vi "Counter_BufferedPulseWidthMeasurement.vi"() -> ()   [LabVIEW 2020]
uses:
  <userlib>/DAQNavi Polymorphic VI/create/DAQNavi Create Channel(Buffered-CI-PulseWidth).vi
  <userlib>/DAQNavi Polymorphic VI/configure/timing/DAQNavi Timing(Buffered Counter Input).vi
  <userlib>/DAQNavi Polymorphic VI/configure/DAQNavi Get Property/CI/DAQNaviGet_Buffered_CI_Record_SectionCount.vi
  <userlib>/DAQNavi Polymorphic VI/read/DAQNavi Read (Buffered Counter Pulse Width).vi
  <userlib>/DAQNavi Polymorphic VI/configure/DAQNavi Get Property/CI/DAQNaviGet_Buffered_CI_Trigger_Level.vi
panel:
  out "data":cluster{"high period":dbl, "low period":dbl}[][](array[cluster])
  out "stopped?":bool
  in  "time out":dbl
  in  "number of samples per channel to read":u32=1000
  out "actual trigger level":dbl
  in  "trigger level":dbl
  out "trigger edge":string
  out "trigger action":string
  out "trigger source":string
  out "sample clock source":string
  in  "section count":i32
  in  "section length":i32
  in  "stop":bool
  out "physical channels":string
  # "Please modify physical channels, sample clock source,  and trigger parameters through DAQNavi Property Assistant VI in block diagram.\nFor this example, when the section count is qual to 0, means the streaming mode for buffered pulse width measurement. Otherwise, means the on buffered mode for buffered pulse width measurement."
  # "Channel Parameters"
  # "Timing Parameters"
  # "Trigger Parameters"
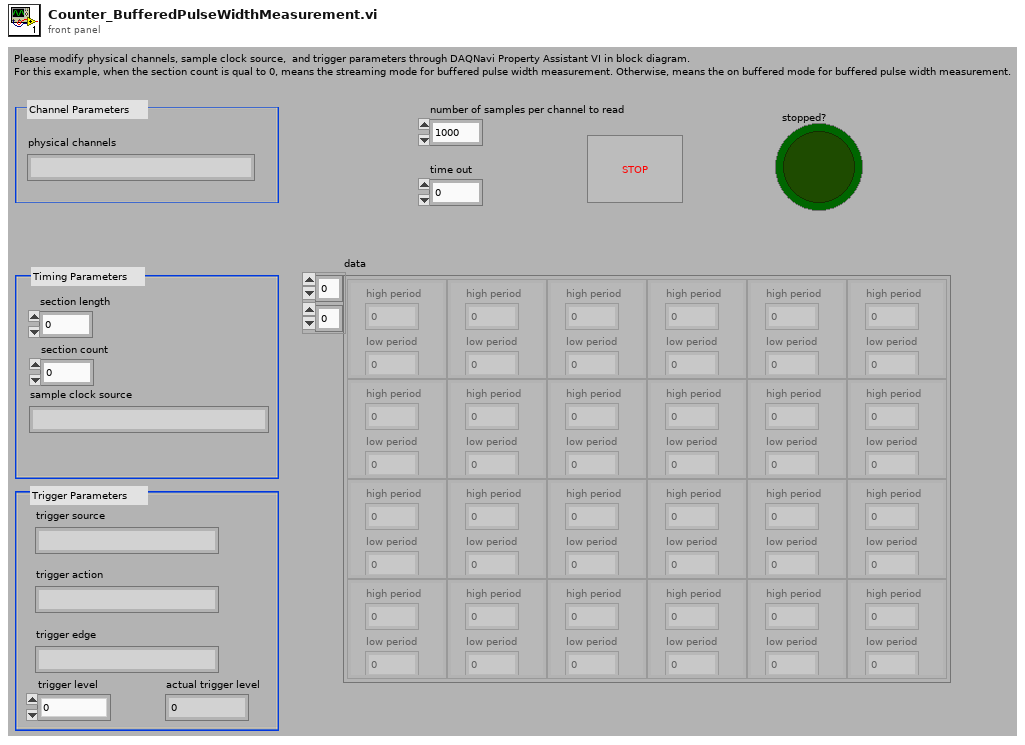
[diagram p1: front panel]
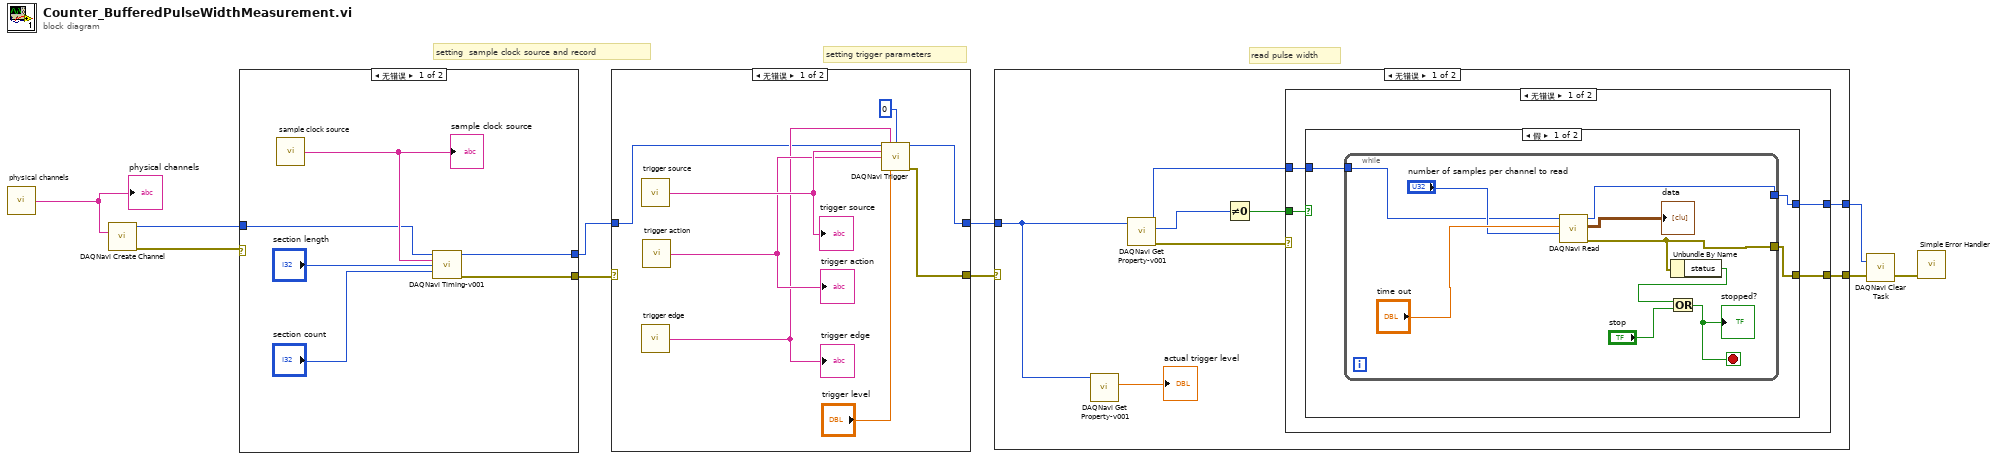
[diagram p0: block diagram]
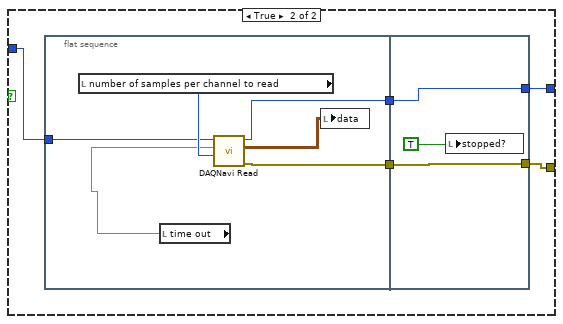
[diagram p2: hidden frame]
diagram:
  # "read pulse width"
  # "setting trigger parameters"
  # "setting  sample clock source and record"
  n1 = call "physical channels"() -> ("property value"=w10:string)  [unwired: 1 out]
  "physical channels" <- w10
  n2 = call-poly <userlib>:"DAQNavi Create Channel.vi"("physical channels"=w10) -> ("task out"=w9:i32, "error out"=w8:errorcluster)  [unwired: 2 in, 11 out]
  n3 = case shown="无错误" w8 {
    selector: w8 -> [_ w17]
    tunnel: w9 -> [w13 w18]
    tunnel: [w12 w18] -> w6
    tunnel: [w11 w17] -> w7
    frame No Error {
      n4 = call "sample clock source"() -> ("property value"=w16:string)  [unwired: 1 out]
      "sample clock source" <- w16
      n5 = call-poly <userlib>:"DAQNavi Timing-v001.vi"("task in"=w13, "sample clock source"=w16, "section length"="section length", "section count"="section count") -> ("task out"=w12:i32, "error out"=w11:errorcluster)  [unwired: 1 in, 9 out]
    }
    frame Error {
    }
  }
  n6 = case shown="无错误" w7 {
    selector: w7 -> [_ w28]
    tunnel: w6 -> [w21 w27]
    tunnel: [w20 w28] -> w5
    tunnel: [w19 w27] -> w4
    frame No Error {
      n7 = call "trigger source"() -> ("property value"=w26:string)  [unwired: 1 out]
      "trigger source" <- w26
      n8 = call "trigger edge"() -> ("property value"=w24:string)  [unwired: 1 out]
      "trigger edge" <- w24
      n9 = call "trigger action"() -> ("property value"=w25:string)  [unwired: 1 out]
      "trigger action" <- w25
      n10 = call <userlib>:"DAQNavi Trigger.vi"("task in"=w21, "edge"=w24, "trigger index"=0, "trigger source"=w26, "action"=w25, "level"="trigger level") -> ("task out"=w19:i32, "error out"=w20:errorcluster)  [unwired: 2 in, 6 out]
    }
    frame Error {
    }
  }
  n11 = case shown="无错误" w5 {
    selector: w5 -> [_ w70]
    tunnel: w4 -> [w35 w69]
    tunnel: [w31 w70] -> w3
    tunnel: [w30 w69] -> w2
    frame No Error {
      n12 = call-poly <userlib>:"DAQNavi Get Property-v001.vi"("task in"=w35) -> ("trigger level"=→"actual trigger level":dbl)  [unwired: 1 in, 9 out]
      n13 = call-poly <userlib>:"DAQNavi Get Property-v001.vi"("task in"=w35) -> ("error out"=w34:errorcluster, "section count"=w33:i32, "task out"=w32:i32)  [unwired: 1 in, 7 out]
      n14 = Not Equal To 0?(x=w33) -> (x != 0?=w29:bool)
      n15 = case shown="无错误" w34 {
        selector: w34 -> [_ w68]
        tunnel: w32 -> [w40 w67]
        tunnel: [w39 w68] -> w31
        tunnel: [w38 w67] -> w30
        tunnel: w29 -> [w37 _]
        frame No Error {
          n16 = case shown="假" w37 {
            tunnel: w40 -> [w43 w57]
            tunnel: [w42 w53] -> w39
            tunnel: [w41 w56] -> w38
            frame False {
              n17 = while {
                tunnel: w43 -> [w50]
                tunnel: [w47] -> w42
                tunnel: [w48] -> w41
                stop <- w45 stop-if-true
                n18 = call-poly <userlib>:"DAQNavi Read.vi"("number of samples per channel to read"="number of samples per channel to read", "timeout"="time out", "task in"=w50) -> ("error out"=w47:errorcluster, "data"=→"data":cluster{"high period":dbl, "low period":dbl}[][], "task out"=w48:i32)  [unwired: 1 in, 5 out]
                n19 = Unbundle By Name(w47) -> ("status"=w46:bool)
                n20 = Or(x=w46, y="stop") -> (x .or. y?=w45:bool)
                "stopped?" <- w45
              }
            }
            frame True {
              n21 = flat-sequence {
                tunnel: w57 -> [w61]
                tunnel: [w60] -> w55
                tunnel: [w59] -> w54
                tunnel: [w65] -> w56
                tunnel: w55 -> [w65]
                tunnel: [w64] -> w53
                tunnel: w54 -> [w64]
                frame #0 {
                  n22 = local read "number of samples per channel to read"() -> (w63:u32)
                  n23 = local read "time out"() -> (w62:dbl)
                  n24 = call-poly <userlib>:"DAQNavi Read.vi"("number of samples per channel to read"=w63, "timeout"=w62, "task in"=w61) -> ("error out"=w59:errorcluster, "data"=w58:cluster{"high period":dbl, "low period":dbl}[][], "task out"=w60:i32)  [unwired: 1 in, 5 out]
                  n25 = local write "data"(w58) -> ()
                }
                frame #1 {
                  n26 = local write "stopped?"(TRUE) -> ()
                }
              }
            }
          }
        }
        frame Error {
        }
      }
    }
    frame Error {
    }
  }
  n27 = call <userlib>:"DAQNavi Clear Task.vi"("error in (no error)"=w3, "task in"=w2) -> ("error out"=w1:errorcluster)  [unwired: 1 out]
  n28 = call <vilib>:"Simple Error Handler.vi"("error in (no error)"=w1) -> ()  [unwired: 1 in, 8 out]
